vi "Create Client from Template.vi"(8 "error in (no error)":errorcluster, 9 "Generated Server Name":string="Generated Server", 10 "Target Project Path":path, 11 "Application ref in":refnum<vi>) -> (0 "error out":errorcluster, 1 "Already exists ?":bool, 2 "Server class out":refnum<vi>, 3 "Server library out":refnum<vi>)   [LabVIEW 2019, in "gRPC Scripting Tools.lvlib"]
uses:
  gRPC Scripting Tools.lvlib
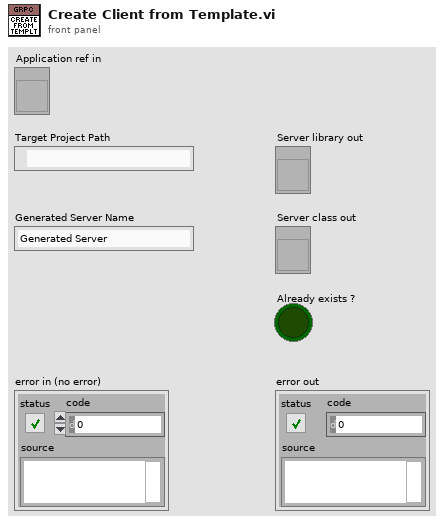
[diagram p1: front panel]
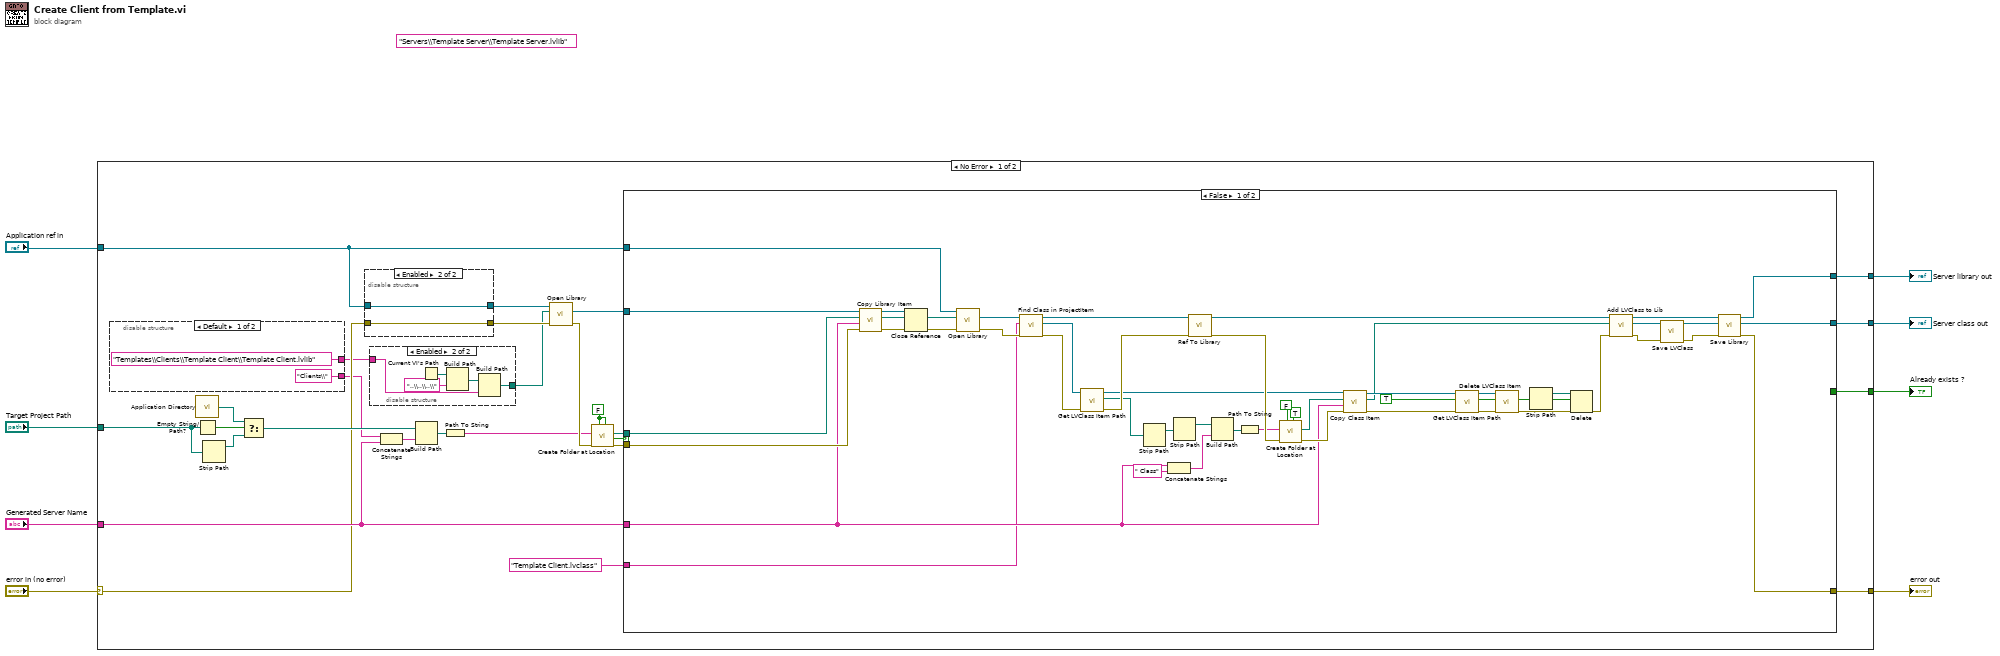
[diagram p0: block diagram]
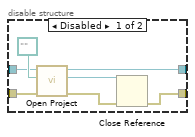
[diagram p2: hidden frame]
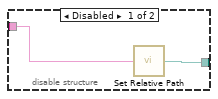
[diagram p3: hidden frame]
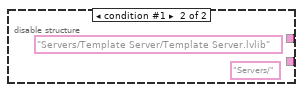
[diagram p4: hidden frame]
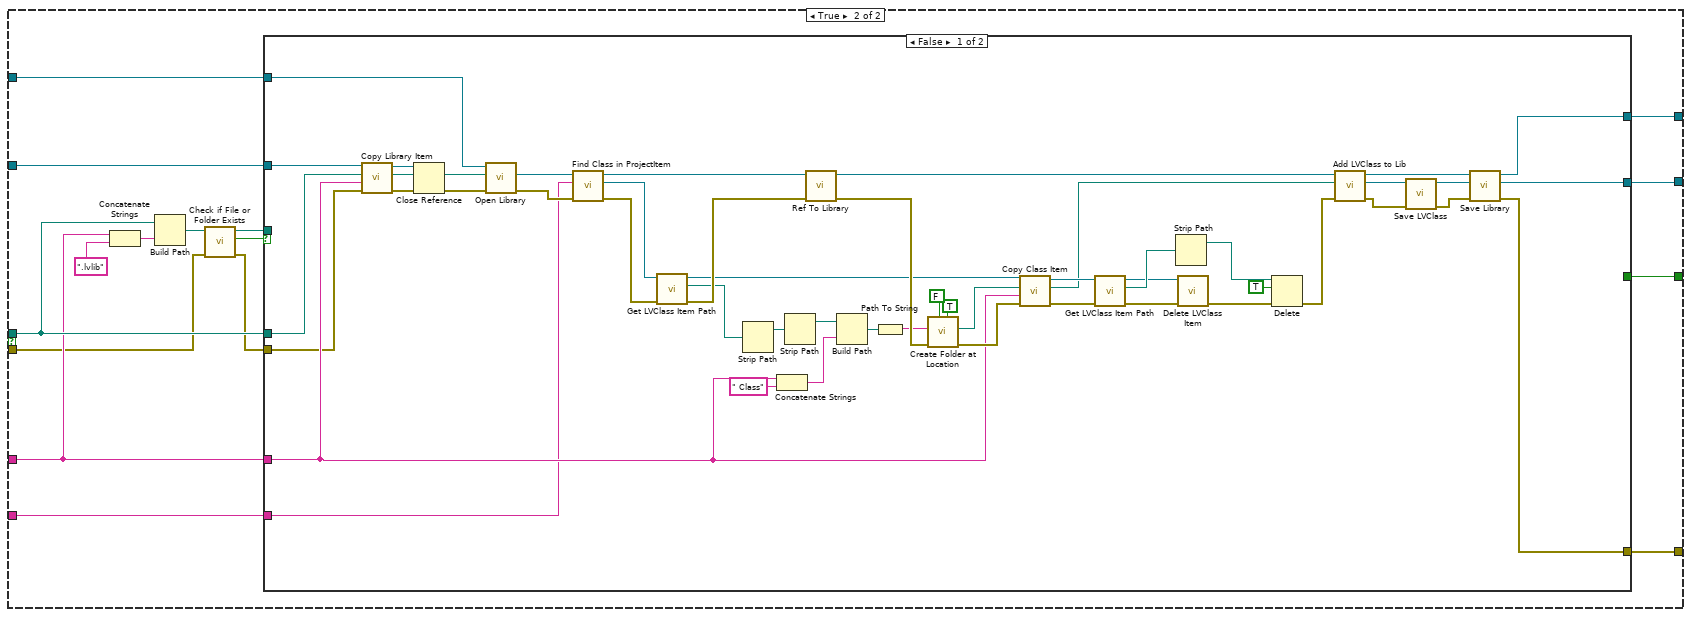
[diagram p5: hidden frame]
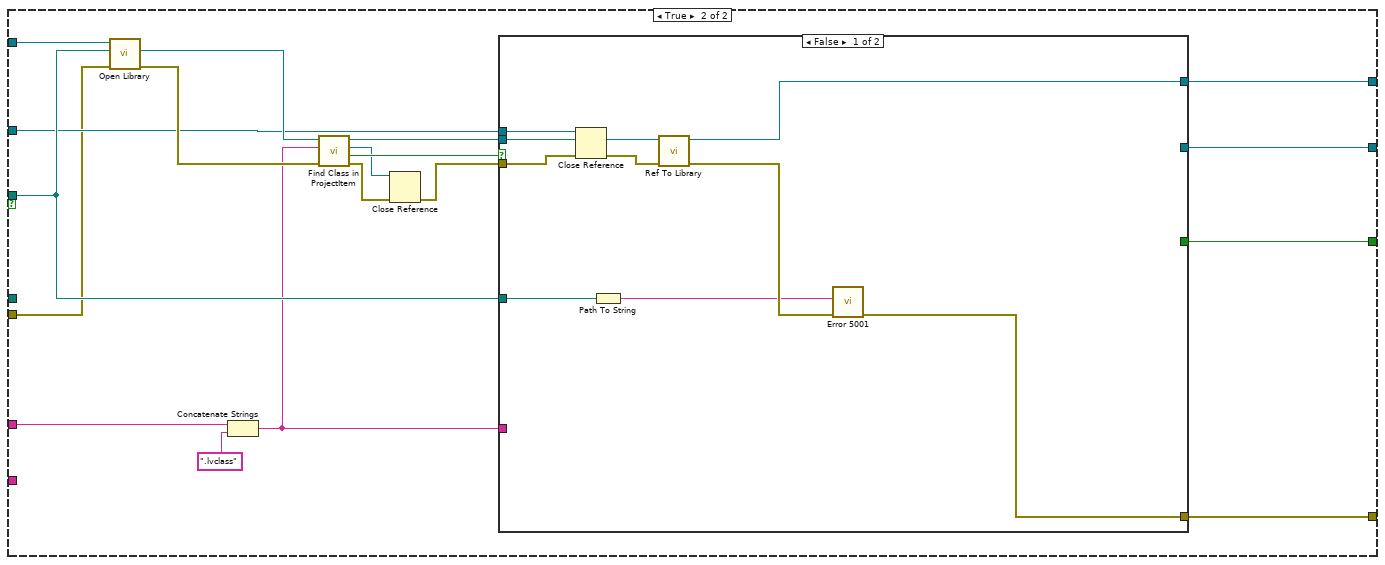
[diagram p6: hidden frame]
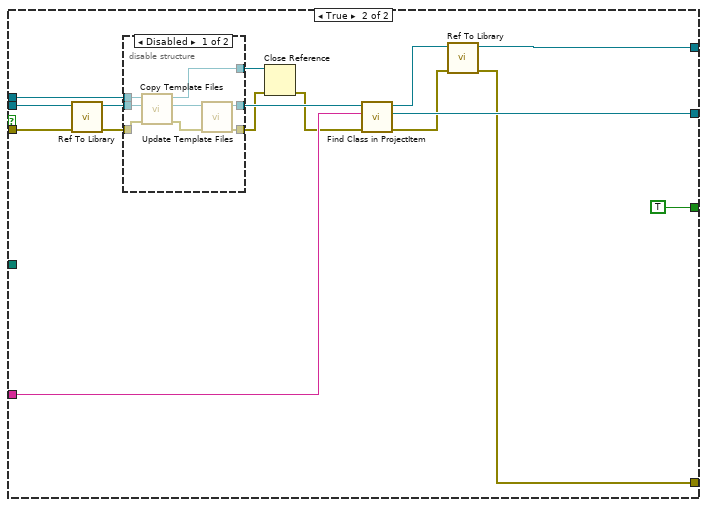
[diagram p7: hidden frame]
diagram:
  (unwired) "Servers\\Template Server\\Template Server.lvlib" ("Application Relative Path")
  n1 = case shown="No Error" "error in (no error)" {
    selector: "error in (no error)" -> [w15 w218]
    tunnel: [w35 w218] -> w8
    tunnel: [w34 _] -> w7
    tunnel: [w33 _] -> w6
    tunnel: "Target Project Path" -> [w18 _]
    tunnel: "Generated Server Name" -> [w17 _]
    tunnel: "Application ref in" -> [w16 _]
    tunnel: [w13 _] -> w1
    frame No Error {
      w27 = FALSE ("Use Relative")
      n2 = disable-structure shown="Default" {
        disable-tunnel: ["Templates\\Clients\\Template Client\\Template Client.lvlib" ("Application Relative Path") _] -> w10
        disable-tunnel: ["Clients\\" ("Path") _] -> w12
        frame condition #0 (active) {
        }
        frame condition #1 {
          (unwired) "Servers/" ("Path")
          (unwired) "Servers/Template Server/Template Server.lvlib" ("Application Relative Path")
        }
      }
      n3 = call <vilib>:"Application Directory.vi"() -> ("Application Directory"=w19:path)
      n4 = Empty String/Path?(string/path=w18) -> (empty?=w22:bool)
      n5 = Strip Path(path=w18) -> (stripped path=w21:path)  [unwired: 1 out]
      n6 = Select(t=w19, s=w22, f=w21) -> (s? t:f=w20:path)
      n7 = disable-structure shown="Enabled" {
        disable-tunnel: [w42 w44] -> w30
        disable-tunnel: [w39 w43] -> w23
        disable-tunnel: w16 -> [w37 w44]
        disable-tunnel: w15 -> [w36 w43]
        frame Disabled {
          n8 = call "Open Project.vi"("error in (no error)"=w36, "Project Path in"=path "", "Application reference"=w37) -> ("error out"=w40:errorcluster, "Project out"=w41:refnum<vi>, "Application out"=w42:refnum<vi>)  [unwired: 6 in]
          n9 = Close Reference(reference=w41, error in (no error)=w40) -> (error out=w39:errorcluster)
        }
        frame Enabled {
        }
      }
      n10 = disable-structure shown="Enabled" {
        disable-tunnel: [w46 w49] -> w9
        disable-tunnel: w10 -> [w45 w47]
        frame Disabled {
          n11 = call "Set Relative Path.vi"("Application Relative Path"=w45) -> ("Full Path"=w46:path)
        }
        frame Enabled {
          n12 = Current VI's Path() -> (path=w51:path)
          n13 = Build Path(base path=w51, name or relative path="..\\..\\..\\") -> (appended path=w48:path)
          n14 = Build Path(base path=w48, name or relative path=w47) -> (appended path=w49:path)
        }
      }
      n15 = Concatenate Strings(w12, w17) -> (w26:string)
      n16 = Build Path(base path=w20, name or relative path=w26) -> (appended path=w25:path)
      n17 = Path To String(path=w25) -> (string=w24:string)
      n18 = call "Open Library.vi"("error in (no error)"=w23, "Full Path"=w9, "Application in"=w30) -> ("error out"=w31:errorcluster, "Library out"=w28:refnum<vi>)  [unwired: 6 in, 1 out]
      n19 = call "Create Folder at Location.vi"("Override existing (F)"=w27, "Use Relative (F)"=w27, "Error In"=w31, "Path"=w24) -> ("Error Out"=w32:errorcluster, "Already Exists ?"=w14:bool, "Full path out"=w29:path)  [unwired: 5 in]
      n20 = case shown="False" w14 {
        tunnel: [w100 w106] -> w35
        tunnel: [w99 w111] -> w34
        tunnel: [w98 w112] -> w33
        tunnel: w32 -> [w63 w103]
        tunnel: w29 -> [w62 w108]
        tunnel: w28 -> [w61 w109]
        tunnel: w17 -> [w56 w107]
        tunnel: w16 -> [w55 w110]
        tunnel: [_ w105] -> w13
        tunnel: "Template Client.lvclass" ("Class Name") -> [w54 w101]
        frame False {
          n21 = call "Copy Library Item.vi"("error in (no error)"=w63, "Copy Name"=w56, "Copy location"=w62, "Library in"=w61) -> ("error out"=w83:errorcluster, "New Lib Path"=w60:path, "Library out"=w82:refnum<vi>)  [unwired: 5 in]
          n22 = Close Reference(reference=w82, error in (no error)=w83) -> (error out=w59:errorcluster)
          n23 = call "Open Library.vi"("error in (no error)"=w59, "Full Path"=w60, "Application in"=w55) -> ("error out"=w57:errorcluster, "Library out"=w58:refnum<vi>)  [unwired: 6 in, 1 out]
          n24 = call "Find Class in ProjectItem.vi"("error in (no error)"=w57, "Class Name"=w54, "ProjectItem in"=w58) -> ("error out"=w65:errorcluster, "LVClass out"=w64:refnum<vi>, "ProjectItem out"=w77:refnum<vi>)  [unwired: 5 in, 1 out]
          n25 = call "Get LVClass Item Path.vi"("error in (no error)"=w65, "LVClassLibrary in"=w64) -> ("error out"=w79:errorcluster, "Path"=w66:path, "LVClassLibrary out"=w67:refnum<vi>)  [unwired: 7 in]
          n26 = Strip Path(path=w66) -> (stripped path=w75:path)  [unwired: 1 out]
          n27 = Concatenate Strings(w56, " Class" ("string")) -> (w70:string)
          n28 = Strip Path(path=w75) -> (stripped path=w76:path)  [unwired: 1 out]
          n29 = call "Ref To Library.vi"("error in (no error)"=w79, "ProjectItem in"=w77) -> ("error out"=w80:errorcluster, "Library out"=w93:refnum<vi>)  [unwired: 8 in]
          n30 = Build Path(base path=w76, name or relative path=w70) -> (appended path=w71:path)
          n31 = Path To String(path=w71) -> (string=w72:string)
          n32 = call "Create Folder at Location.vi"("Override existing (F)"=TRUE, "Use Relative (F)"=FALSE ("Use Relative"), "Error In"=w80, "Path"=w72) -> ("Error Out"=w81:errorcluster, "Full path out"=w74:path)  [unwired: 5 in, 1 out]
          n33 = call "Copy Class Item.vi"("error in (no error)"=w81, "New Name"=w56, "Full path in"=w74, "LVClassLibrary in"=w67) -> ("error out"=w85:errorcluster, "New Class Path out"=w78:path, "LVClassLibrary out"=w84:refnum<vi>)  [unwired: 5 in]
          n34 = call "Get LVClass Item Path.vi"("error in (no error)"=w85, "LVClassLibrary in"=w84) -> ("error out"=w87:errorcluster, "Path"=w88:path, "LVClassLibrary out"=w86:refnum<vi>)  [unwired: 7 in]
          n35 = call "Delete LVClass Item.vi"("error in (no error)"=w87, "LVClassLibrary in"=w86) -> ("error out"=w90:errorcluster)  [unwired: 9 in]
          n36 = Strip Path(path=w88) -> (stripped path=w89:path)  [unwired: 1 out]
          n37 = Delete(path (use dialog)=w89, entire hierarchy (F)=TRUE, error in=w90) -> (error out=w91:errorcluster)  [unwired: 2 in, 2 out]
          n38 = call "Add LVClass to Lib.vi"("error in (no error)"=w91, "LVClass Path in"=w78, "Library in"=w93) -> ("error out"=w96:errorcluster, "LVClassLibrary out"=w95:refnum<vi>, "Library out"=w94:refnum<vi>)  [unwired: 6 in]
          n39 = call "Save LVClass.vi"("error in (no error)"=w96, "LVClassLibrary in"=w95) -> ("error out"=w97:errorcluster, "LVClassLibrary out"=w99:refnum<vi>)  [unwired: 8 in]
          n40 = call "Save Library.vi"("error in (no error)"=w97, "Library in"=w94) -> ("error out"=w100:errorcluster, "Library out"=w98:refnum<vi>)  [unwired: 8 in]
        }
        frame True {
          n41 = Concatenate Strings(w107, ".lvlib" ("string")) -> (w115:string)
          n42 = Build Path(base path=w108, name or relative path=w115) -> (appended path=w114:path)
          n43 = call <vilib>:"Check if File or Folder Exists.vi"("error in (no error)"=w103, "path"=w114) -> ("error out"=w102:errorcluster, "file or folder exists?"=w113:bool, "dup path"=w104:path)  [unwired: 7 in]
          n44 = case shown="False" w113 {
            tunnel: [w125 w175] -> w112
            tunnel: [w124 w164] -> w111
            tunnel: w110 -> [w123 w181]
            tunnel: w109 -> [w122 w170]
            tunnel: w108 -> [w121 _]
            tunnel: w107 -> [w120 w179]
            tunnel: w102 -> [w119 w169]
            tunnel: [w118 w174] -> w106
            tunnel: [_ w172] -> w105
            tunnel: w104 -> [_ w171]
            tunnel: w101 -> [w117 _]
            frame False {
              n45 = call "Copy Library Item.vi"("error in (no error)"=w119, "Copy Name"=w120, "Copy location"=w121, "Library in"=w122) -> ("error out"=w149:errorcluster, "New Lib Path"=w129:path, "Library out"=w148:refnum<vi>)  [unwired: 5 in]
              n46 = Close Reference(reference=w148, error in (no error)=w149) -> (error out=w128:errorcluster)
              n47 = call "Open Library.vi"("error in (no error)"=w128, "Full Path"=w129, "Application in"=w123) -> ("error out"=w126:errorcluster, "Library out"=w127:refnum<vi>)  [unwired: 6 in, 1 out]
              n48 = call "Find Class in ProjectItem.vi"("error in (no error)"=w126, "Class Name"=w117, "ProjectItem in"=w127) -> ("error out"=w131:errorcluster, "LVClass out"=w130:refnum<vi>, "ProjectItem out"=w143:refnum<vi>)  [unwired: 5 in, 1 out]
              n49 = call "Get LVClass Item Path.vi"("error in (no error)"=w131, "LVClassLibrary in"=w130) -> ("error out"=w145:errorcluster, "Path"=w132:path, "LVClassLibrary out"=w133:refnum<vi>)  [unwired: 7 in]
              n50 = Strip Path(path=w132) -> (stripped path=w141:path)  [unwired: 1 out]
              n51 = Concatenate Strings(w120, " Class" ("string")) -> (w136:string)
              n52 = Strip Path(path=w141) -> (stripped path=w142:path)  [unwired: 1 out]
              n53 = call "Ref To Library.vi"("error in (no error)"=w145, "ProjectItem in"=w143) -> ("error out"=w146:errorcluster, "Library out"=w159:refnum<vi>)  [unwired: 8 in]
              n54 = Build Path(base path=w142, name or relative path=w136) -> (appended path=w137:path)
              n55 = Path To String(path=w137) -> (string=w138:string)
              n56 = call "Create Folder at Location.vi"("Override existing (F)"=TRUE, "Use Relative (F)"=FALSE ("Use Relative"), "Error In"=w146, "Path"=w138) -> ("Error Out"=w147:errorcluster, "Full path out"=w140:path)  [unwired: 5 in, 1 out]
              n57 = call "Copy Class Item.vi"("error in (no error)"=w147, "New Name"=w120, "Full path in"=w140, "LVClassLibrary in"=w133) -> ("error out"=w151:errorcluster, "New Class Path out"=w144:path, "LVClassLibrary out"=w150:refnum<vi>)  [unwired: 5 in]
              n58 = call "Get LVClass Item Path.vi"("error in (no error)"=w151, "LVClassLibrary in"=w150) -> ("error out"=w153:errorcluster, "Path"=w154:path, "LVClassLibrary out"=w152:refnum<vi>)  [unwired: 7 in]
              n59 = Strip Path(path=w154) -> (stripped path=w155:path)  [unwired: 1 out]
              n60 = call "Delete LVClass Item.vi"("error in (no error)"=w153, "LVClassLibrary in"=w152) -> ("error out"=w156:errorcluster)  [unwired: 9 in]
              n61 = Delete(path (use dialog)=w155, entire hierarchy (F)=TRUE, error in=w156) -> (error out=w157:errorcluster)  [unwired: 2 in, 2 out]
              n62 = call "Add LVClass to Lib.vi"("error in (no error)"=w157, "LVClass Path in"=w144, "Library in"=w159) -> ("error out"=w162:errorcluster, "LVClassLibrary out"=w161:refnum<vi>, "Library out"=w160:refnum<vi>)  [unwired: 6 in]
              n63 = call "Save LVClass.vi"("error in (no error)"=w162, "LVClassLibrary in"=w161) -> ("error out"=w163:errorcluster, "LVClassLibrary out"=w124:refnum<vi>)  [unwired: 8 in]
              n64 = call "Save Library.vi"("error in (no error)"=w163, "Library in"=w160) -> ("error out"=w118:errorcluster, "Library out"=w125:refnum<vi>)  [unwired: 8 in]
            }
            frame True {
              n65 = call "Open Library.vi"("error in (no error)"=w169, "Full Path"=w171, "Application in"=w181) -> ("error out"=w177:errorcluster, "Library out"=w180:refnum<vi>)  [unwired: 6 in, 1 out]
              n66 = Concatenate Strings(w179, ".lvclass" ("Class Name")) -> (w165:string)
              n67 = call "Find Class in ProjectItem.vi"("error in (no error)"=w177, "Class Name"=w165, "ProjectItem in"=w180) -> ("error out"=w167:errorcluster, "Found?"=w173:bool, "LVClass out"=w168:refnum<vi>, "ProjectItem out"=w176:refnum<vi>)  [unwired: 5 in]
              n68 = Close Reference(reference=w168, error in (no error)=w167) -> (error out=w166:errorcluster)
              n69 = case shown="False" w173 {
                tunnel: w176 -> [w190 w201]
                tunnel: [w189 w206] -> w175
                tunnel: w166 -> [w184 w203]
                tunnel: [w187 w194] -> w174
                tunnel: w171 -> [w186 _]
                tunnel: [_ TRUE] -> w172
                tunnel: w170 -> [w185 w193]
                tunnel: w165 -> [_ w200]
                tunnel: [_ w199] -> w164
                frame False {
                  n70 = Close Reference(reference=w185, error in (no error)=w184) -> (error out=w183:errorcluster)
                  n71 = Path To String(path=w186) -> (string=w182:string)
                  n72 = call "Ref To Library.vi"("error in (no error)"=w183, "ProjectItem in"=w190) -> ("error out"=w188:errorcluster, "Library out"=w189:refnum<vi>)  [unwired: 8 in]
                  n73 = call "Error 5001.vi"("error in (no error)"=w188, "Server Class Path"=w182) -> ("error out"=w187:errorcluster)  [unwired: 9 in]
                }
                frame True {
                  n74 = call "Ref To Library.vi"("error in (no error)"=w203, "ProjectItem in"=w201) -> ("error out"=w202:errorcluster, "Library out"=w204:refnum<vi>)  [unwired: 8 in]
                  n75 = disable-structure shown="Disabled" {
                    disable-tunnel: w204 -> [w214 w216]
                    disable-tunnel: w202 -> [w213 w215]
                    disable-tunnel: [w212 w216] -> w198
                    disable-tunnel: w193 -> [w211 w217]
                    disable-tunnel: [w208 w215] -> w192
                    disable-tunnel: [w207 w217] -> w191
                    frame Disabled {
                      n76 = call "Copy Template Files.vi"("error in (no error)"=w213, "Server Library (Library Item) in"=w214, "Template Library (Library Item) in"=w211) -> ("error out"=w210:errorcluster, "Server Library (Library Item) out"=w209:refnum<vi>, "Template Library (Library Item) out"=w207:refnum<vi>)  [unwired: 6 in]
                      n77 = call "Update Template Files.vi"("error in (no error)"=w210, "Server Library (Library Item) in"=w209) -> ("error out"=w208:errorcluster, "Server Library (Library Item) out"=w212:refnum<vi>)  [unwired: 8 in]
                    }
                    frame Enabled {
                    }
                  }
                  n78 = Close Reference(reference=w191, error in (no error)=w192) -> (error out=w196:errorcluster)
                  n79 = call "Find Class in ProjectItem.vi"("error in (no error)"=w196, "Class Name"=w200, "ProjectItem in"=w198) -> ("error out"=w195:errorcluster, "LVClass out"=w199:refnum<vi>, "ProjectItem out"=w197:refnum<vi>)  [unwired: 5 in, 1 out]
                  n80 = call "Ref To Library.vi"("error in (no error)"=w195, "ProjectItem in"=w197) -> ("error out"=w194:errorcluster, "Library out"=w206:refnum<vi>)  [unwired: 8 in]
                }
              }
            }
          }
        }
      }
    }
    frame Error {
    }
  }
  "error out" <- w8
  "Server class out" <- w7
  "Server library out" <- w6
  "Already exists ?" <- w1
